vi "AdaptToInputs.vi"(0 "XRef":T8, 1 "Term Types":T5, 2 "State In":T1) -> (14 "Reply":T3, 15 "Fatal Error Out":T2, 16 "State Out":T1)   [LabVIEW 2015, in "LVJSON.lvlib" / "Set Object Parameters.xnode"]
uses:
  Set Object Parameters.xnode
  <vilib>/XNodeSupport/XNodeXNodeRef.ctl
  <vilib>/XNodeSupport/XNodeTermTypeIDPairs.ctl
  <vilib>/XNodeSupport/XNodeTermTypeIDPair.ctl
  <vilib>/XNodeSupport/XNodeType.ctl
  <vilib>/XNodeSupport/XNodeString.ctl
  State.ctl
  <vilib>/XNodeSupport/XNodeStringArray.ctl
  <vilib>/XNodeSupport/XNodeErrorCluster.ctl
  <vilib>/Utility/Data Type/NI_Data Type.lvlib
  <vilib>/XNodeSupport/NI_XNodeSupport.lvlib
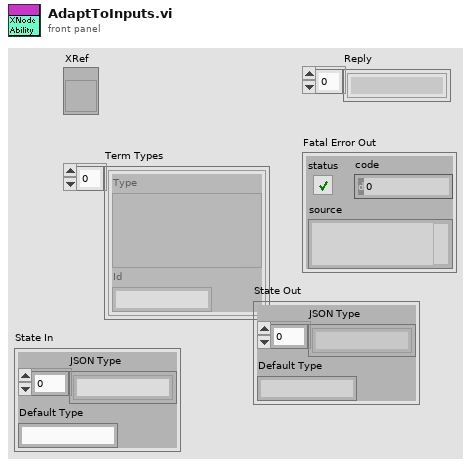
[diagram p1: front panel]
types:
  T1 = typedef "LVJSON.lvlib/Set Object Parameters.xnode/State.ctl" = cluster{"JSON Type":string[], "Default Type":string}
  T2 = typedef "NI_XNodeSupport.lvlib/XNodeErrorCluster.ctl" = errorcluster
  T3 = typedef "NI_XNodeSupport.lvlib/XNodeStringArray.ctl" = T4[]
  T4 = typedef "NI_XNodeSupport.lvlib/XNodeString.ctl" = string
  T5 = typedef "NI_XNodeSupport.lvlib/XNodeTermTypeIDPairs.ctl" = T6[]
  T6 = typedef "NI_XNodeSupport.lvlib/XNodeTermTypeIDPair.ctl" = cluster{"Type":T7, "Id":T4}
  T7 = typedef "NI_XNodeSupport.lvlib/XNodeType.ctl" = variant
  T8 = typedef "NI_XNodeSupport.lvlib/XNodeXNodeRef.ctl" = refnum<vi>
  T9 = typedef "NI_Data Type.lvlib/Data Type.ctl" = enum8{"Invalid Type", "Void", "I8", "I16", "I32", "I64", "U8", "U16", "U32", "U64", "Single Float", "Double Float", "Extended Float", "Single Complex", "Double Complex", "Extended Complex", "Enum U8", "Enum U16", "Enum U32", "Enum U64", "Single Float With Unit", "Double Float With Unit", "Extended Float With Unit", "Single Complex with Unit", "Double Complex with Unit", "Extended Complex with Unit", "Boolean", "String", "Path", "Picture", "Tag", "Array", "Cluster", "Variant", "LV Variant", "Waveform", "Timestamp", "Digital Waveform", "Digital Data", "ExpressData", "Refnum", "External Data", "VI", "Poly VI", "LabVIEW Class Instance", "Fixed Point"}
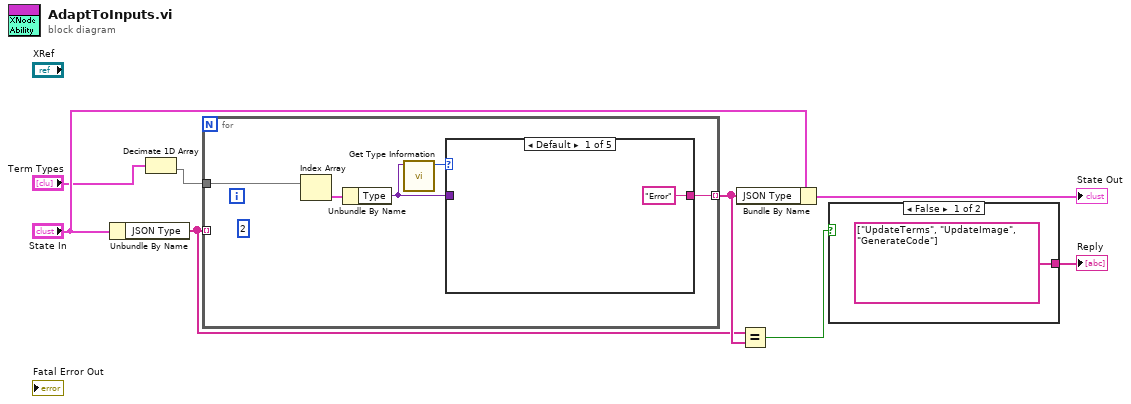
[diagram p0: block diagram]
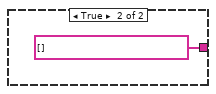
[diagram p2: hidden frame]
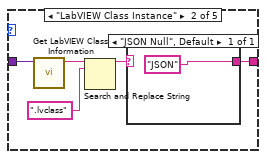
[diagram p3: hidden frame]
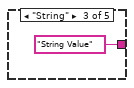
[diagram p4: hidden frame]
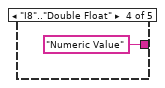
[diagram p5: hidden frame]
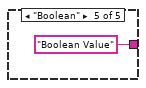
[diagram p6: hidden frame]
diagram:
  n1 = Unbundle By Name("State In") -> ("JSON Type"=w3:string[])
  n2 = Decimate 1D Array("Term Types") -> (w1:T6[])  [unwired: 1 out]
  n3 = for {
    tunnel: w3 -> [_] mode=indexing
    tunnel: w1 -> [w13]
    tunnel: [w9] -> w5 mode=indexing
    (unwired) 2 ("y")
    n4 = Index Array(array=w13) -> (element=w12:T6)  [unwired: 1 in]
    n5 = Unbundle By Name(w12) -> ("Type"=w10:T7)
    n6 = call <vilib>:"Get Type Information.vi"("Variant"=w10) -> ("Type"=w11:T9)  [unwired: 6 in, 4 out]
    n7 = case shown="Default" w11 {
      tunnel: w10 -> [_ w19 _ _ _]
      tunnel: ["Error" w15 "String Value" "Numeric Value" "Boolean Value"] -> w9
      frame Default {
      }
      frame "LabVIEW Class Instance" {
        n8 = call <vilib>:"Get LabVIEW Class Information.vi"("Variant"=w19) -> ("LabVIEW Class File Name"=w18:string)  [unwired: 8 in, 2 out]
        n9 = Search and Replace String(input string=w18, search string=".lvclass") -> (result string=w16:string)  [unwired: 6 in, 3 out]
        n10 = case shown="\"JSON Null\", Default" w16 {
          tunnel: ["JSON"] -> w15
          frame "JSON Null", Default {
          }
        }
      }
      frame "String" {
      }
      frame "I8".."Double Float" {
      }
      frame "Boolean" {
      }
    }
  }
  n11 = Bundle By Name(cluster="State In", "JSON Type"=w5) -> (→"State Out":T1)
  n12 = Equal?(x=w3, y=w5) -> (x = y?=w4:bool)
  n13 = case shown="False" w4 {
    tunnel: [T3 ["UpdateTerms", "UpdateImage", "GenerateCode"] ("Reply") T3 [] ("Reply")] -> w6
    frame False {
    }
    frame True {
    }
  }
  "Reply" <- w6
